vi "XNET TCP Socket Close.vi"(8 "error in":errorcluster, 10 "abort (F)":bool, 11 "socket":refnum<k20>) -> (0 "error out":errorcluster)   [LabVIEW 2018]
doc: "Closes a TCP network connection."
uses:
  nixlvapi.dll
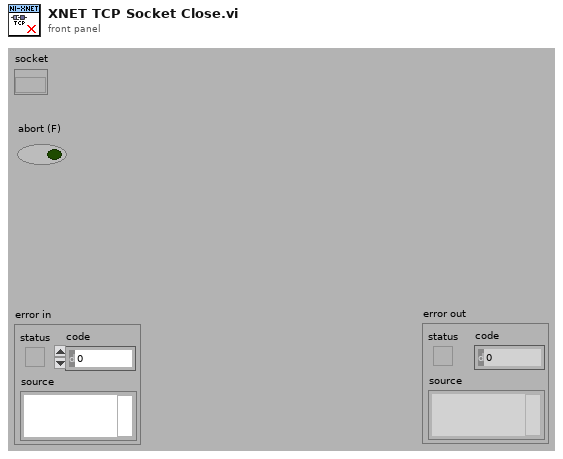
[diagram p1: front panel]
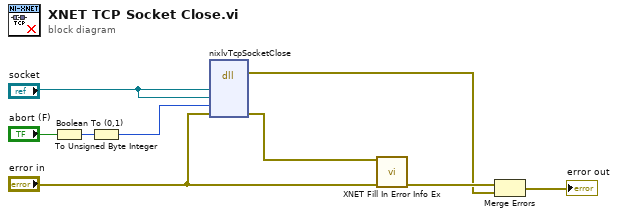
[diagram p0: block diagram]
diagram:
  n1 = Boolean To (0,1)(Boolean="abort (F)") -> (0, 1=w3:i16)
  n2 = To Unsigned Byte Integer(number=w3) -> (unsigned 8bit integer=w1:u8)
  n3 = dll-call lib="nixlvapi.*" fn="nixlvTcpSocketClose" label="Call Library"("socketRef"="socket", "socketRefObjPtr"="socket", "abort"=w1, "errorInOut"="error in") -> (error out=w7:errorcluster, "errorInOut"=w9:errorcluster)  [unwired: 3 in, 5 out]
  n4 = call "XNET Fill In Error Info Ex.vi"("error xnet"=w9, "error in"="error in") -> ("error out"=w8:errorcluster)  [unwired: 13 in]
  n5 = Merge Errors(w8, w7) -> (→"error out":errorcluster)
